vi "Fit Result to String.vi"(8 "error in (no error)":errorcluster, 11 "Sinusoidal Fit in":refnum<class "Sinusoidal Fit.lvclass">) -> (0 "error out":errorcluster, 2 "Array":string[](array[string]), 3 "Sinusoidal Fit out":refnum<class "Sinusoidal Fit.lvclass">)   [LabVIEW 2016, in "Sinusoidal Fit.lvclass"]
uses:
  Sinusoidal Fit.lvclass
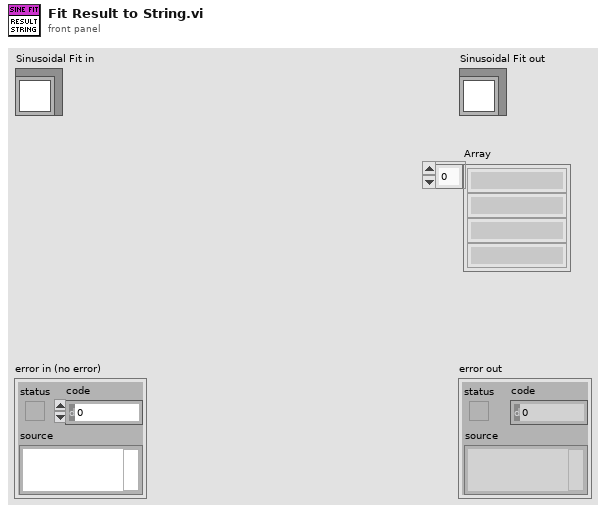
[diagram p1: front panel]
types:
  T1 = typedef "Typedef - Gain and Phase.ctl" = cluster{"Gain":dbl, "Gain SD":dbl, "Phase":dbl, "Phase SD":dbl}
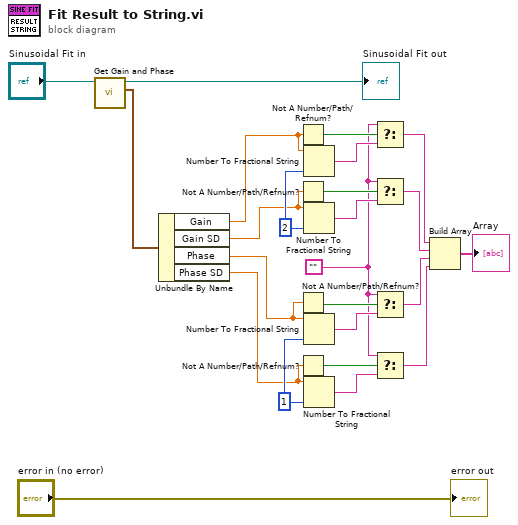
[diagram p0: block diagram]
diagram:
  w1 = ""
  w19 = i16 1 ("precision (6)")
  w20 = i16 2 ("precision (6)")
  n1 = call-dynamic "Get Gain and Phase.vi"("Sinusoidal Fit in"="Sinusoidal Fit in") -> ("Gain and Phase"=w21:T1, "Sinusoidal Fit out"=→"Sinusoidal Fit out":refnum<class "Sinusoidal Fit.lvclass">)  [unwired: 8 in, 1 out]
  n2 = Unbundle By Name(w21) -> ("Gain"=w3:dbl, "Gain SD"=w7:dbl, "Phase"=w16:dbl, "Phase SD"=w11:dbl)
  n3 = Not A Number/Path/Refnum?(number/path/refnum=w3) -> (NaN/Path/Refnum?=w2:bool)
  n4 = Not A Number/Path/Refnum?(number/path/refnum=w7) -> (NaN/Path/Refnum?=w6:bool)
  n5 = Not A Number/Path/Refnum?(number/path/refnum=w16) -> (NaN/Path/Refnum?=w17:bool)
  n6 = Not A Number/Path/Refnum?(number/path/refnum=w11) -> (NaN/Path/Refnum?=w10:bool)
  n7 = Number To Fractional String(number=w3, precision (6)=w20) -> (F-format string=w5:string)  [unwired: 2 in]
  n8 = Number To Fractional String(number=w7, precision (6)=w20) -> (F-format string=w9:string)  [unwired: 2 in]
  n9 = Number To Fractional String(number=w16, precision (6)=w19) -> (F-format string=w15:string)  [unwired: 2 in]
  n10 = Number To Fractional String(number=w11, precision (6)=w19) -> (F-format string=w13:string)  [unwired: 2 in]
  n11 = Select(t=w1, s=w2, f=w5) -> (s? t:f=w4:string)
  n12 = Select(t=w1, s=w6, f=w9) -> (s? t:f=w8:string)
  n13 = Select(t=w1, s=w17, f=w15) -> (s? t:f=w14:string)
  n14 = Select(t=w1, s=w10, f=w13) -> (s? t:f=w12:string)
  n15 = Build Array(w4, w8, w14, w12) -> (→"Array":string[])
  "error out" <- "error in (no error)"
